vi "Analog Input.vi"(6 "clai. Parmeter":T1, 8 "error in":errorcluster, 9 "Min Value":string[](array[string]), 10 "Max Value":string[](array[string]), 11 "DAQmx Analog Input Setting":T2={"DAQmx Analog Input_00"="Dev1/ai0", "DAQmx Analog Input_01"="Dev1/ai1", "DAQmx Analog Input_02"="Dev1/ai2", "DAQmx Analog Input_03"="Dev1/ai3", "DAQmx Analog Input_04"="Dev1/ai4", "DAQmx Analog Input_05"="Dev1/ai5", "DAQmx Analog Input_06"="Dev1/ai6", "DAQmx Analog Input_07"="Dev1/ai7", "DAQmx Analog Input_00 2"="Dev1/ai8", "DAQmx Analog Input_01 2"="Dev1/ai9", "DAQmx Analog Input_02 2"="Dev1/ai10", "DAQmx Analog Input_03 2"="Dev1/ai11", "DAQmx Analog Input_04 2"="Dev1/ai12", "DAQmx Analog Input_05 2"="Dev1/ai13", "DAQmx Analog Input_06 2"="Dev1/ai14", "DAQmx Analog Input_07 2"="Dev1/ai15", "DAQmx Analog Input_00 3"="Dev1/ai16", "DAQmx Analog Input_01 3"="Dev1/ai17", "DAQmx Analog Input_02 3"="Dev1/ai18", "DAQmx Analog Input_03 3"="Dev1/ai19", "DAQmx Analog Input_04 3"="Dev1/ai20", "DAQmx Analog Input_05 3"="Dev1/ai21", "DAQmx Analog Input_06 3"="Dev1/ai22", "DAQmx Analog Input_07 3"="Dev1/ai23", "DAQmx Analog Input_00 4"="Dev1/ai24", "DAQmx Analog Input_01 4"="Dev1/ai25", "DAQmx Analog Input_02 4"="Dev1/ai26", "DAQmx Analog Input_03 4"="Dev1/ai27", "DAQmx Analog Input_04 4"="Dev1/ai28", "DAQmx Analog Input_05 4"="Dev1/ai29", "DAQmx Analog Input_06 4"="Dev1/ai30", "DAQmx Analog Input_07 4"="Dev1/ai31"}) -> (0 "error out":errorcluster, 1 "Exit":bool)   [LabVIEW 2015]
uses:
  <vilib>/DAQmx/read.llb/DAQmx Read (Analog 2D DBL NChan NSamp).vi
  <vilib>/Analysis/baseanly.llb/Mean (DBL).vi
  <vilib>/DAQmx/create/channels.llb/DAQmx Create Channel (AI-Voltage-Basic).vi
  <vilib>/DAQmx/configure/timing.llb/DAQmx Timing (Sample Clock).vi
  Galobal variable_TI.vi
  <vilib>/DAQmx/miscellaneous.llb/DAQmx Fill In Error Info.vi
  <vilib>/Analysis/NI_AALBase.lvlib
panel:
  out "data":dbl[][](array[numeric])
  in  "error in 2":errorcluster
  out "error out 4":errorcluster
  out "x-y 2":u32
  out "error out 3":errorcluster
  out "Exit  2":bool
  in  "Max Value 2":string[](array[string])
  in  "Min Value 2":string[](array[string])
  in  "clai. Parmeter 2":T1
  out "x-y":u32
  out "error out 2":errorcluster
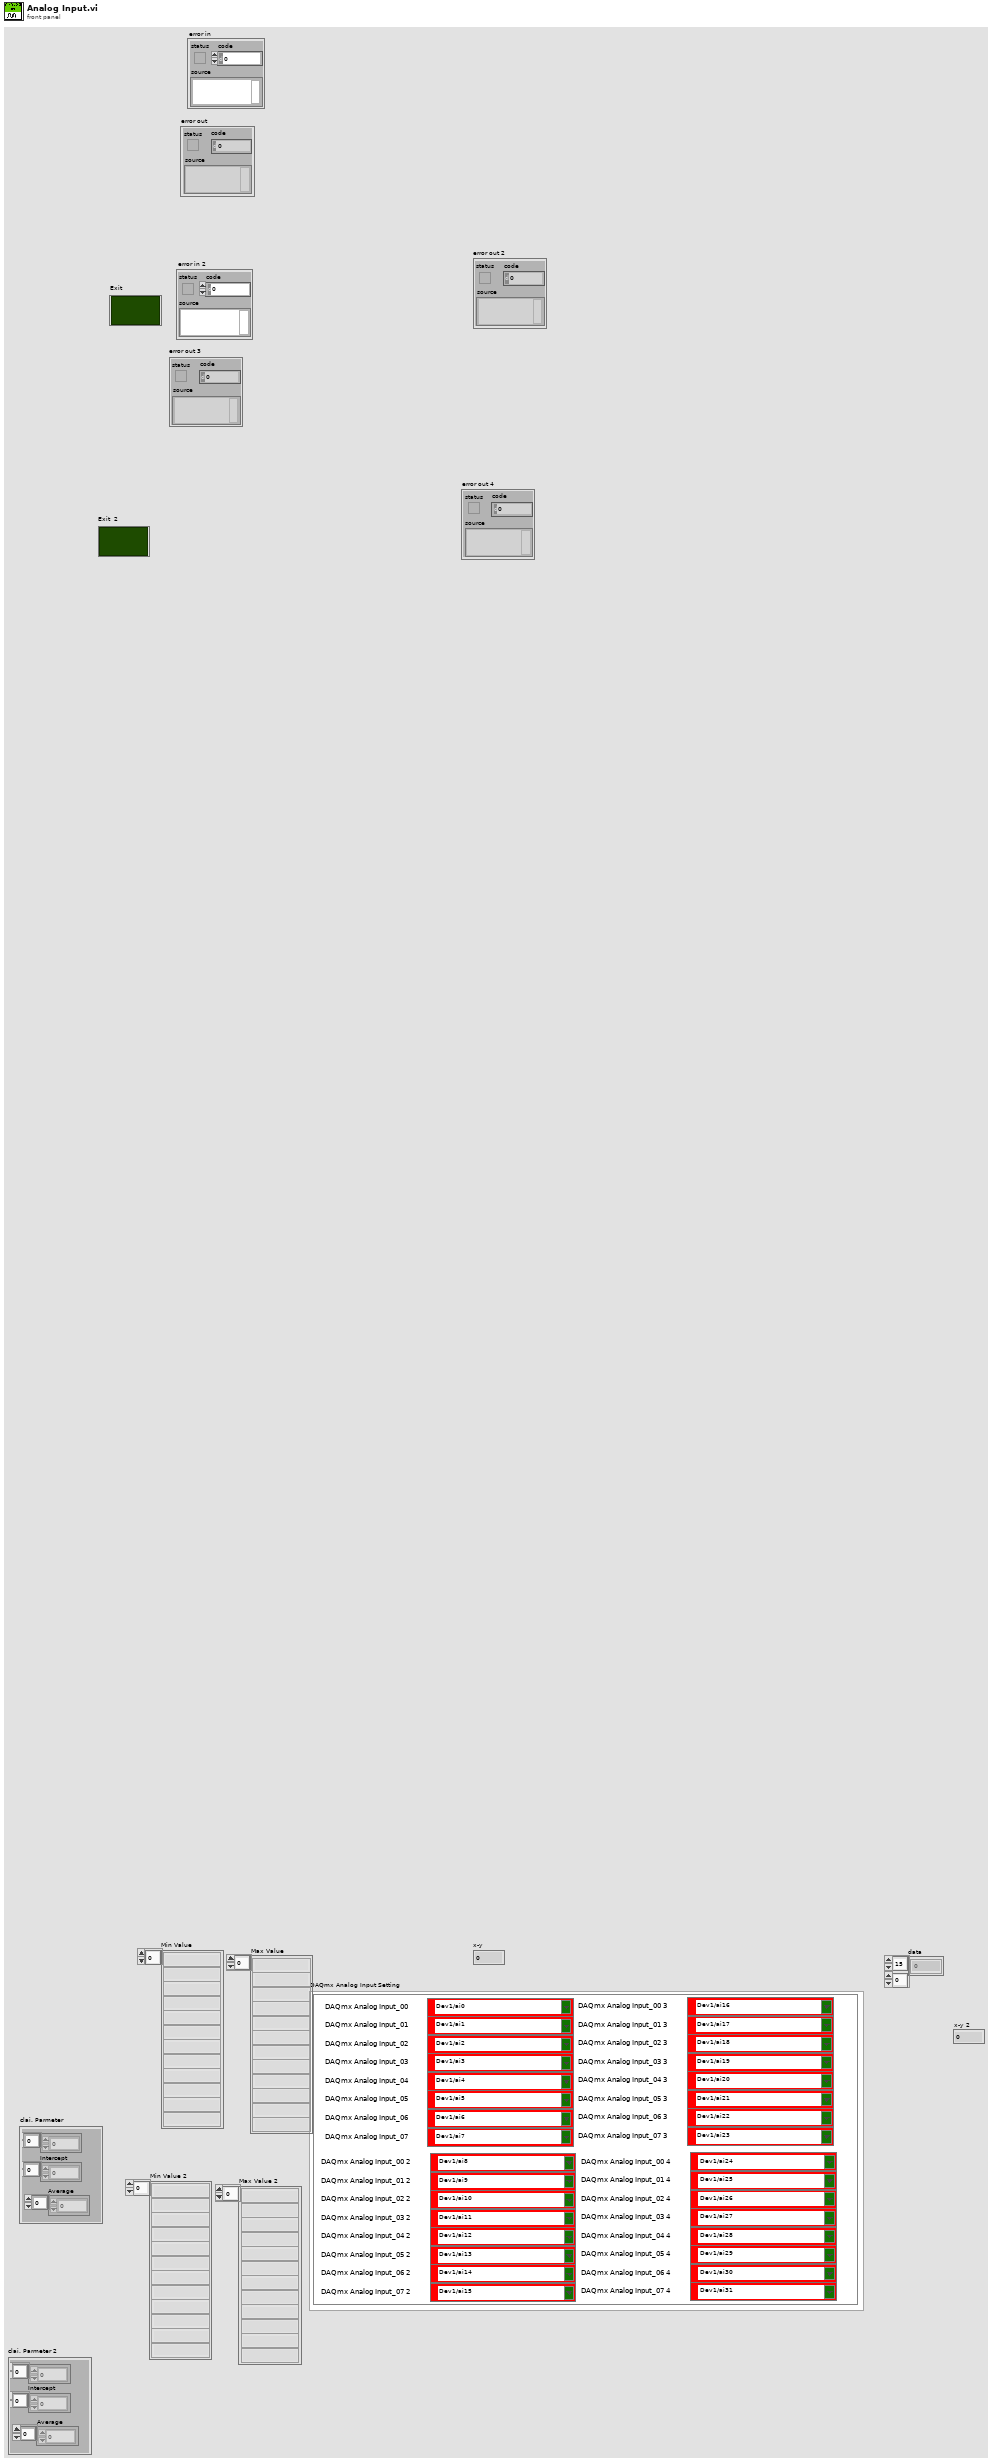
[diagram p1: front panel]
types:
  T1 = cluster{"Slop":dbl[], "Intercept":dbl[], "Average ":i16[]}
  T2 = cluster{"DAQmx Analog Input_00":tag, "DAQmx Analog Input_01":tag, "DAQmx Analog Input_02":tag, "DAQmx Analog Input_03":tag, "DAQmx Analog Input_04":tag, "DAQmx Analog Input_05":tag, "DAQmx Analog Input_06":tag, "DAQmx Analog Input_07":tag, "DAQmx Analog Input_00 2":tag, "DAQmx Analog Input_01 2":tag, "DAQmx Analog Input_02 2":tag, "DAQmx Analog Input_03 2":tag, "DAQmx Analog Input_04 2":tag, "DAQmx Analog Input_05 2":tag, "DAQmx Analog Input_06 2":tag, "DAQmx Analog Input_07 2":tag, "DAQmx Analog Input_00 3":tag, "DAQmx Analog Input_01 3":tag, "DAQmx Analog Input_02 3":tag, "DAQmx Analog Input_03 3":tag, "DAQmx Analog Input_04 3":tag, "DAQmx Analog Input_05 3":tag, "DAQmx Analog Input_06 3":tag, "DAQmx Analog Input_07 3":tag, "DAQmx Analog Input_00 4":tag, "DAQmx Analog Input_01 4":tag, "DAQmx Analog Input_02 4":tag, "DAQmx Analog Input_03 4":tag, "DAQmx Analog Input_04 4":tag, "DAQmx Analog Input_05 4":tag, "DAQmx Analog Input_06 4":tag, "DAQmx Analog Input_07 4":tag}
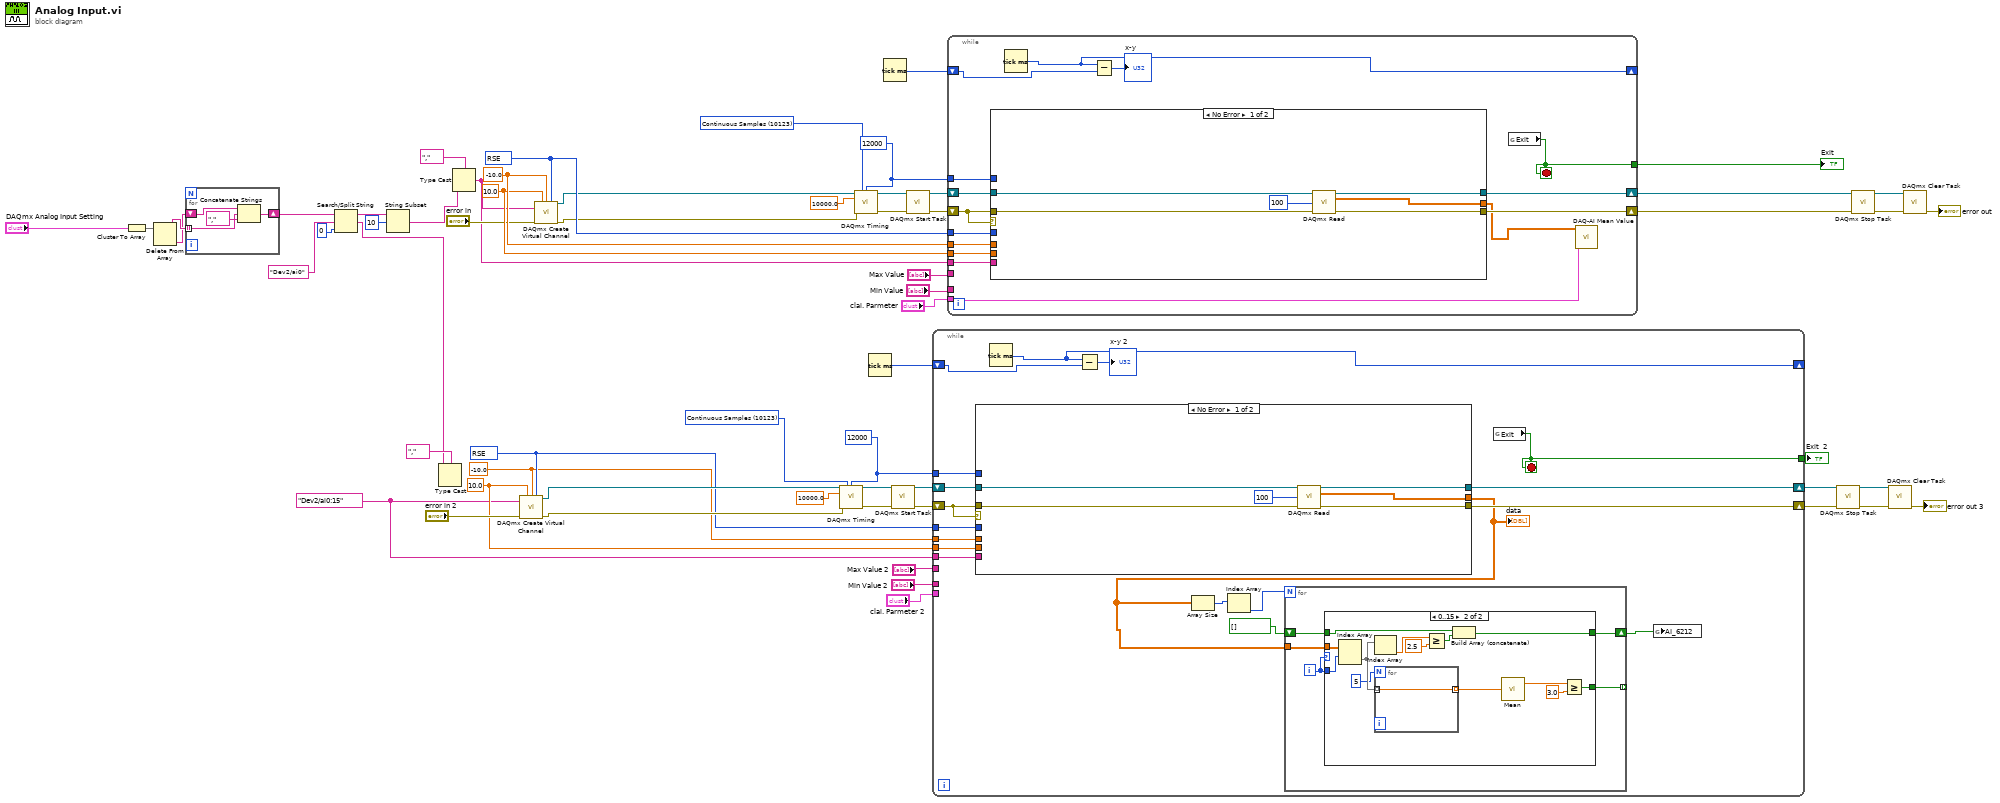
[diagram p0: block diagram]
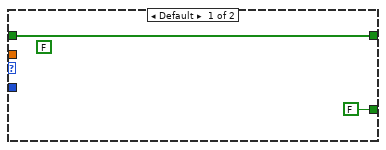
[diagram p2: hidden frame]
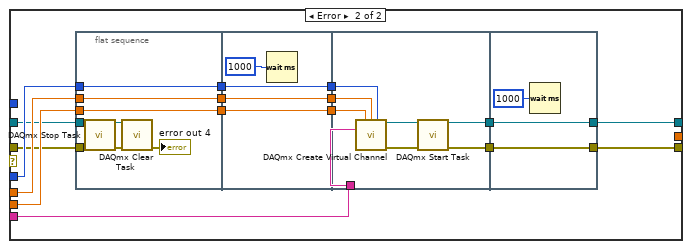
[diagram p3: hidden frame]
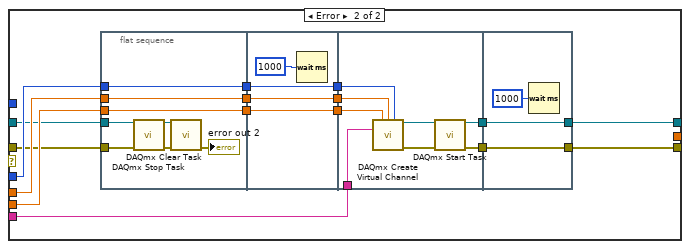
[diagram p4: hidden frame]
diagram:
  w1 = tag "Dev2/ai0:15" ("physical channels")
  w23 = 12000 ("samples per channel")
  w16 = 10123 items=["Finite Samples"=10178, "Continuous Samples"=10123, "Hardware Timed Single Point"=12522] ("sample mode")
  w12 = 10083 items=["default"=-1, "RSE"=10083, "NRSE"=10078, "Differential"=10106, "Pseudodifferential"=12529] ("input terminal configuration")
  w10 = -10.0 ("minimum value")
  w11 = 10.0 ("maximum value")
  w42 = 12000 ("samples per channel")
  w55 = 10123 items=["Finite Samples"=10178, "Continuous Samples"=10123, "Hardware Timed Single Point"=12522] ("sample mode")
  w59 = 10083 items=["default"=-1, "RSE"=10083, "NRSE"=10078, "Differential"=10106, "Pseudodifferential"=12529] ("input terminal configuration")
  w61 = -10.0 ("minimum value")
  w60 = 10.0 ("maximum value")
  n1 = Cluster To Array(cluster="DAQmx Analog Input Setting") -> (array=w52:tag[])
  n2 = Delete From Array(array=w52) -> (deleted portion=w50:tag, array with subset deleted=w51:tag[])  [unwired: 2 in]
  n3 = for {
    tunnel: w51 -> [w65] mode=indexing
    shift-right: [w63] -> w7
    shift-left: w50 -> [w62]
    n4 = Concatenate Strings(w62, tag "," ("1."), w65) -> (w63:string)
  }
  n5 = Search/Split String(string=w7, search string/char (-)="Dev2/ai0", offset (0)=0) -> (substring before match=w5:string, match + rest of string=w2:string)  [unwired: 1 out]
  n6 = String Subset(string=w5, offset (0)=10) -> (substring=w3:string)  [unwired: 1 in]
  n7 = Type Cast(type=tag "," ("1."), x=w2) -> ()  [unwired: 1 out]
  n8 = Type Cast(type=tag "," ("1."), x=w3) -> (*(type *) &x=w53:tag)
  n9 = call-poly <vilib>:"DAQmx Create Virtual Channel.vi"("maximum value"=w11, "minimum value"=w10, "input terminal configuration"=w12, "physical channels"=w1, "error in"="error in 2") -> ("task out"=w31:refnum<k21>, "error out"=w32:errorcluster)  [unwired: 4 in, 5 out]
  n10 = call-poly <vilib>:"DAQmx Create Virtual Channel.vi"("maximum value"=w60, "minimum value"=w61, "input terminal configuration"=w59, "physical channels"=w53, "error in"="error in") -> ("task out"=w34:refnum<k21>, "error out"=w33:errorcluster)  [unwired: 4 in, 5 out]
  n11 = call-poly <vilib>:"DAQmx Timing.vi"("task/channels in"=w31, "sample mode"=w16, "samples per channel"=w23, "rate"=10000.0, "error in"=w32) -> ("task out"=w14:refnum<k21>, "error out"=w15:errorcluster)  [unwired: 9 in]
  n12 = call-poly <vilib>:"DAQmx Timing.vi"("task/channels in"=w34, "sample mode"=w55, "samples per channel"=w42, "rate"=10000.0, "error in"=w33) -> ("task out"=w57:refnum<k21>, "error out"=w56:errorcluster)  [unwired: 9 in]
  n13 = Tick Count (ms)() -> (millisecond timer value=w24:u32)
  n14 = Tick Count (ms)() -> (millisecond timer value=w41:u32)
  n15 = call <vilib>:"DAQmx Start Task.vi"("task/channels in"=w14, "error in"=w15) -> ("task out"=w18:refnum<k21>, "error out"=w19:errorcluster)  [unwired: 12 out]
  n16 = call <vilib>:"DAQmx Start Task.vi"("task/channels in"=w57, "error in"=w56) -> ("task out"=w47:refnum<k21>, "error out"=w46:errorcluster)  [unwired: 12 out]
  n17 = while {
    shift-right: [w80] -> w20
    shift-left: w19 -> [w83]
    shift-right: [w81] -> w21
    shift-left: w18 -> [w82]
    tunnel: w1 -> [w79]
    tunnel: w10 -> [w78]
    tunnel: w11 -> [w77]
    tunnel: w12 -> [w76]
    tunnel: [w75] -> w22
    tunnel: w23 -> [w74]
    shift-right: [w72] -> _
    shift-left: w24 -> [w73]
    tunnel: "Max Value 2" -> [_]
    tunnel: "Min Value 2" -> [_]
    tunnel: "clai. Parmeter 2" -> [_]
    stop <- w75 stop-if-true
    n18 = case shown="No Error" w83 {
      tunnel: w83 -> [w109 w113]
      tunnel: w82 -> [w110 w114]
      tunnel: [w108 w112] -> w81
      tunnel: [w107 w111] -> w80
      tunnel: w79 -> [_ w126]
      tunnel: w78 -> [_ w125]
      tunnel: w77 -> [_ w124]
      tunnel: w76 -> [_ w123]
      tunnel: [w106 _] -> w68
      tunnel: w74 -> [_ _]
      frame No Error {
        n19 = call-poly <vilib>:"DAQmx Read.vi"("task/channels in"=w110, "number of samples per channel"=100, "error in"=w109) -> ("task out"=w108:refnum<k21>, "data"=w106:dbl[][], "error out"=w107:errorcluster)  [unwired: 10 out]
      }
      frame Error {
        n20 = flat-sequence {
          tunnel: w123 -> [w132]
          tunnel: w124 -> [w133]
          tunnel: w125 -> [w134]
          tunnel: [w134] -> w117
          tunnel: [w133] -> w116
          tunnel: [w132] -> w115
          tunnel: w114 -> [w130]
          tunnel: w113 -> [w129]
          tunnel: [w138] -> w120
          tunnel: [w137] -> w119
          tunnel: [w136] -> w118
          tunnel: w117 -> [w138]
          tunnel: w116 -> [w137]
          tunnel: w115 -> [w136]
          tunnel: w126 -> [w144]
          tunnel: [w140] -> w122
          tunnel: [w139] -> w121
          tunnel: w120 -> [w143]
          tunnel: w119 -> [w142]
          tunnel: w118 -> [w141]
          tunnel: [w148] -> w111
          tunnel: [w149] -> w112
          tunnel: w122 -> [w149]
          tunnel: w121 -> [w148]
          frame #0 {
            n21 = call <vilib>:"DAQmx Stop Task.vi"("task/channels in"=w130, "error in"=w129) -> ("task out"=w127:refnum<k21>, "error out"=w131:errorcluster)  [unwired: 12 in]
            n22 = call <vilib>:"DAQmx Clear Task.vi"("task in"=w127, "error in"=w131) -> ("error out"=→"error out 4":errorcluster)  [unwired: 13 in]
          }
          frame #1 {
            n23 = Wait (ms)(milliseconds to wait=u32 1000) -> ()  [unwired: 1 out]
          }
          frame #2 {
            n24 = call-poly <vilib>:"DAQmx Create Virtual Channel.vi"("maximum value"=w142, "minimum value"=w143, "input terminal configuration"=w141, "physical channels"=w144) -> ("task out"=w146:refnum<k21>, "error out"=w145:errorcluster)  [unwired: 5 in, 5 out]
            n25 = call <vilib>:"DAQmx Start Task.vi"("task/channels in"=w146, "error in"=w145) -> ("task out"=w140:refnum<k21>, "error out"=w139:errorcluster)  [unwired: 12 out]
          }
          frame #3 {
            n26 = Wait (ms)(milliseconds to wait=u32 1000) -> ()  [unwired: 1 out]
          }
        }
      }
    }
    "data" <- w68
    n27 = Tick Count (ms)() -> (millisecond timer value=w72:u32)
    n28 = Subtract(x=w72, y=w73) -> (x-y=→"x-y 2":u32)
    n29 = Array Size(array=w68) -> (size(s)=w69:i32[])
    n30 = Index Array(array=w69) -> (element=w67:i32)  [unwired: 1 in]
    n31 = for {
      N: w67 -> [_]
      tunnel: w68 -> [w88]
      tunnel: [w87] -> _ mode=indexing
      shift-right: [w85] -> w66
      shift-left: bool[] [] -> [w84]
      i -> [w86]
      n32 = case shown="0..15" w86 {
        tunnel: w88 -> [_ w103]
        tunnel: w86 -> [_ w94]
        tunnel: [FALSE w95] -> w87
        tunnel: [w89 w92] -> w85
        tunnel: w84 -> [w89 w91]
        frame Default {
          (unwired) FALSE
        }
        frame 0..15 {
          n33 = Index Array(array=w103, index (row)=w94) -> (element=w100:dbl[])  [unwired: 1 in]
          n34 = Index Array(array=w100) -> (element=w102:dbl)  [unwired: 1 in]
          n35 = for {
            N: 5 -> [_]
            tunnel: w100 -> [w104] mode=indexing
            tunnel: [w104] -> w98 mode=indexing
          }
          n36 = Greater Or Equal?(x=w102, y=2.5) -> (x >= y?=w93:bool)
          n37 = Build Array (concatenate)(w91, w93) -> (w92:bool[])
          n38 = call-poly <vilib>:"Mean.vi"("X"=w98) -> ("mean"=w96:dbl)  [unwired: 1 out]
          n39 = Greater Or Equal?(x=w96, y=3.0) -> (x >= y?=w95:bool)
        }
      }
    }
    n40 = global read "Galobal variable_TI.vi" "Exit"() -> (w75:bool)
    n41 = global write "Galobal variable_TI.vi" "AI_6212"(w66) -> ()
  }
  "Exit  2" <- w22
  n42 = while {
    shift-right: [w161] -> w45
    shift-left: w46 -> [w164]
    shift-right: [w162] -> w44
    shift-left: w47 -> [w163]
    tunnel: w53 -> [w160]
    tunnel: w61 -> [w159]
    tunnel: w60 -> [w158]
    tunnel: w59 -> [w157]
    tunnel: [w156] -> w43
    tunnel: w42 -> [w155]
    shift-right: [w153] -> _
    shift-left: w41 -> [w154]
    tunnel: "Max Value" -> [_]
    tunnel: "Min Value" -> [_]
    tunnel: "clai. Parmeter" -> [w151]
    stop <- w156 stop-if-true
    n43 = case shown="No Error" w164 {
      tunnel: w164 -> [w169 w173]
      tunnel: w163 -> [w170 w174]
      tunnel: [w168 w172] -> w162
      tunnel: [w167 w171] -> w161
      tunnel: w160 -> [_ w186]
      tunnel: w159 -> [_ w185]
      tunnel: w158 -> [_ w184]
      tunnel: w157 -> [_ w183]
      tunnel: [w166 _] -> w150
      tunnel: w155 -> [_ _]
      frame No Error {
        n44 = call-poly <vilib>:"DAQmx Read.vi"("task/channels in"=w170, "number of samples per channel"=100, "error in"=w169) -> ("task out"=w168:refnum<k21>, "data"=w166:dbl[][], "error out"=w167:errorcluster)  [unwired: 10 out]
      }
      frame Error {
        n45 = flat-sequence {
          tunnel: w183 -> [w192]
          tunnel: w184 -> [w193]
          tunnel: w185 -> [w194]
          tunnel: [w194] -> w177
          tunnel: [w193] -> w176
          tunnel: [w192] -> w175
          tunnel: w174 -> [w190]
          tunnel: w173 -> [w189]
          tunnel: [w198] -> w180
          tunnel: [w197] -> w179
          tunnel: [w196] -> w178
          tunnel: w177 -> [w198]
          tunnel: w176 -> [w197]
          tunnel: w175 -> [w196]
          tunnel: w186 -> [w204]
          tunnel: [w200] -> w182
          tunnel: [w199] -> w181
          tunnel: w180 -> [w203]
          tunnel: w179 -> [w202]
          tunnel: w178 -> [w201]
          tunnel: [w208] -> w171
          tunnel: [w209] -> w172
          tunnel: w182 -> [w209]
          tunnel: w181 -> [w208]
          frame #0 {
            n46 = call <vilib>:"DAQmx Stop Task.vi"("task/channels in"=w190, "error in"=w189) -> ("task out"=w187:refnum<k21>, "error out"=w191:errorcluster)  [unwired: 12 in]
            n47 = call <vilib>:"DAQmx Clear Task.vi"("task in"=w187, "error in"=w191) -> ("error out"=→"error out 2":errorcluster)  [unwired: 13 in]
          }
          frame #1 {
            n48 = Wait (ms)(milliseconds to wait=u32 1000) -> ()  [unwired: 1 out]
          }
          frame #2 {
            n49 = call-poly <vilib>:"DAQmx Create Virtual Channel.vi"("maximum value"=w202, "minimum value"=w203, "input terminal configuration"=w201, "physical channels"=w204) -> ("task out"=w206:refnum<k21>, "error out"=w205:errorcluster)  [unwired: 5 in, 5 out]
            n50 = call <vilib>:"DAQmx Start Task.vi"("task/channels in"=w206, "error in"=w205) -> ("task out"=w200:refnum<k21>, "error out"=w199:errorcluster)  [unwired: 12 out]
          }
          frame #3 {
            n51 = Wait (ms)(milliseconds to wait=u32 1000) -> ()  [unwired: 1 out]
          }
        }
      }
    }
    n52 = Tick Count (ms)() -> (millisecond timer value=w153:u32)
    n53 = Subtract(x=w153, y=w154) -> (x-y=→"x-y":u32)
    n54 = global read "Galobal variable_TI.vi" "Exit"() -> (w156:bool)
    n55 = call "DAQ-AI Mean Value.vi"("Cluster"=w151, "data"=w150) -> ()  [unwired: 9 in, 1 out]
  }
  "Exit" <- w43
  n56 = call <vilib>:"DAQmx Stop Task.vi"("task/channels in"=w21, "error in"=w20) -> ("task out"=w27:refnum<k21>, "error out"=w28:errorcluster)  [unwired: 12 in]
  n57 = call <vilib>:"DAQmx Stop Task.vi"("task/channels in"=w44, "error in"=w45) -> ("task out"=w38:refnum<k21>, "error out"=w37:errorcluster)  [unwired: 12 in]
  n58 = call <vilib>:"DAQmx Clear Task.vi"("task in"=w27, "error in"=w28) -> ("error out"=→"error out 3":errorcluster)  [unwired: 13 in]
  n59 = call <vilib>:"DAQmx Clear Task.vi"("task in"=w38, "error in"=w37) -> ("error out"=→"error out":errorcluster)  [unwired: 13 in]
